vi "Calibrate.vi"(8 "error in (no error)":errorcluster, 11 "VISA resource name":refnum<visa-resource-name>) -> (0 "error out":errorcluster, 2 "Calibration Result":bool, 3 "VISA resource name out":refnum<visa-resource-name>)   [LabVIEW 2014, in "Agilent U2000 Series.lvlib"]
doc: "Performs calibration on the specified channel."
uses:
  Agilent U2000 Series.lvlib
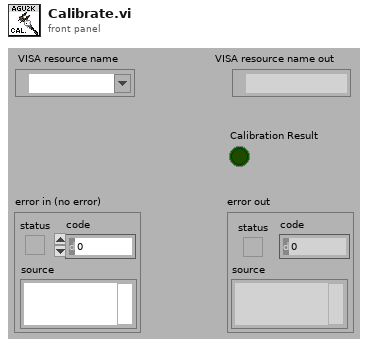
[diagram p1: front panel]
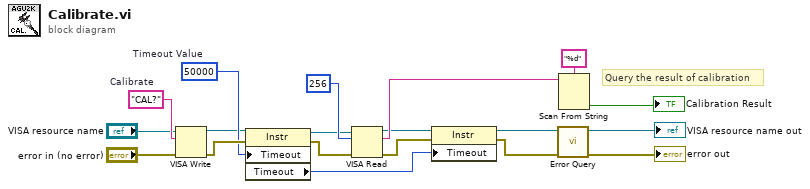
[diagram p0: block diagram]
diagram:
  w6 = u32 50000  # Timeout Value
  w18 = "CAL?"  # Calibrate
  # "Query the result of calibration"
  n1 = VISA Write(VISA resource name="VISA resource name", write buffer=w18, error in (no error)="error in (no error)") -> (VISA resource name out=w5:refnum<visa-resource-name>, error out=w12:errorcluster)  [unwired: 1 out]
  n2 = property class="Instr"(reference=w5, error in=w12, "Timeout"=w6) -> (reference out=w8:refnum<visa-resource-name>, error out=w7:errorcluster, "Timeout"=w9:u32)
  n3 = VISA Read(VISA resource name=w8, byte count=u32 256, error in (no error)=w7) -> (VISA resource name out=w11:refnum<visa-resource-name>, read buffer=w16:string, error out=w10:errorcluster)  [unwired: 1 out]
  n4 = property class="Instr"(reference=w11, error in=w10, "Timeout"=w9) -> (reference out=w3:refnum<visa-resource-name>, error out=w4:errorcluster)
  n5 = call "Error Query.vi"("error in (no error)"=w4, "VISA resource name"=w3) -> ("error out"=→"error out":errorcluster, "VISA resource name out"=→"VISA resource name out":refnum<visa-resource-name>)  [unwired: 8 out]
  n6 = Scan From String(format string="%d", input string=w16) -> (output 1=→"Calibration Result":bool)  [unwired: 2 in, 4 out]
